vi "Write coeffs.vi"(8 "error in (no error)":errorcluster, 10 "coeffs":dbl[][](array[numeric]), 11 "Polynomial Scale configuration in":refnum<class "Polynomial Scale configuration.lvclass">) -> (0 "error out":errorcluster, 3 "Polynomial Scale configuration out":refnum<class "Polynomial Scale configuration.lvclass">)   [LabVIEW 2013]
uses:
  Polynomial Scale configuration.lvclass
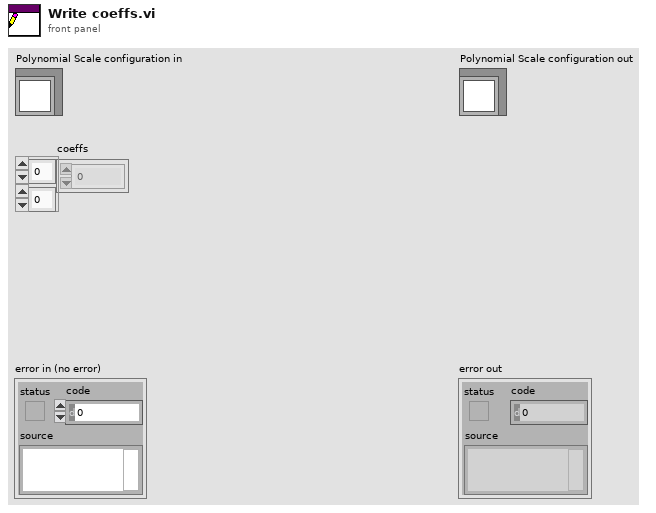
[diagram p1: front panel]
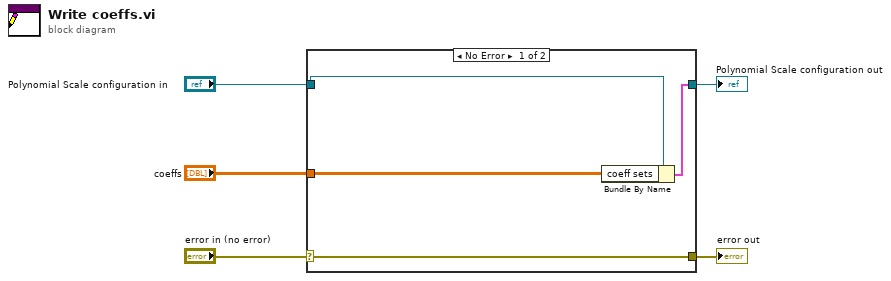
[diagram p0: block diagram]
diagram:
  n1 = case shown="No Error" "error in (no error)" {
    selector: "error in (no error)" -> [w9 w10]
    tunnel: [w9 w10] -> w4
    tunnel: [w7 w11] -> w2
    tunnel: "Polynomial Scale configuration in" -> [w8 w11]
    tunnel: "coeffs" -> [w6 _]
    frame No Error {
      n2 = Bundle By Name(cluster=w8, "coeff sets"=w6) -> (w7:cluster{})
    }
    frame Error {
    }
  }
  "error out" <- w4
  "Polynomial Scale configuration out" <- w2
